vi "Test UI-Bus U32 Vars.vi"() -> ()   [LabVIEW 2021]
uses:
  Source/UI-Bus/UI-Bus.lvclass
  C:/Program Files (x86)/National Instruments/LabVIEW 2021/vi.lib/TSA/Omni-Bus/Omni-Bus/Bus Access/Bus_Access.lvclass
  <vilib>/TSA/Omni-Bus/Omni-Bus/Omni_Bus.lvclass
  <vilib>/TSA/Omni-Bus/Omni-Bus/Support/Broad Types.ctl
  <vilib>/Utility/Data Type/Type Definitions/Data Type.ctl
  <vilib>/TSA/Abstract Data Classes/Abs_Types/Type/Abs_Type.lvclass/Abs_Type.ctl
  <vilib>/TSA/Omni-Bus/Omni-Bus/Omni_Bus.lvclass/Omni_Bus.ctl
  <vilib>/TSA/Omni-Bus/Omni-Bus/Support/Read/Read Multi U32.vi
  <vilib>/TSA/Omni-Bus/Omni-Bus/Support/Write/Write U32.vi
  <vilib>/TSA/Omni-Bus/Omni-Bus/Support/Get/Get Multi U32.vi
  <vilib>/TSA/Omni-Bus/Omni-Bus/Support/FindVar.vi
  <vilib>/TSA/Omni-Bus/Omni-Bus/Support/FindMultiVar.vi
  <vilib>/Utility/error.llb/Clear Errors.vi
  <vilib>/TSA/Omni-Bus/Omni-Bus/Properties/Read Var Map.vi
  <vilib>/TSA/Abstract Data Classes/Abs_Types/Type/Properties/Read Tag.vi
  <vilib>/TSA/Abstract Data Classes/Abs_Types/U32 Integer/Abs_U32 Integer.lvclass
  C:/Program Files (x86)/National Instruments/LabVIEW 2021/vi.lib/TSA/Abstract Data Classes/Abs_Types/Type/Abs_Type.lvclass
  <vilib>/TSA/Abstract Data Classes/Abs_Types/Value/Abs_Value.lvclass
  <vilib>/TSA/Omni-Bus/Omni-Bus/Support/Check For Read Only Error.vi
  <vilib>/TSA/Omni-Bus/Omni-Bus/Support/Incorrect Tag String Error.vi
  <vilib>/TSA/Abstract Data Classes/Abs_Types/Type/Abs_Type.lvclass
  <vilib>/Utility/Data Type/NI_Data Type.lvlib
panel:
  in  "Tab Control":enum32{"Page 1", "Page 2"}(tab)
  out "Gauge":u32(knob) scale=0.0..10.0
  out "Tank":u32(slide) scale=0.0..10.0
  out "Thermometer":u32(slide) scale=0.0..100.0
  in  "Dial":u32(knob) scale=0.0..10.0
  out "Meter":u32(knob) scale=0.0..10.0
  in  "Knob":u32(knob) scale=0.0..10.0
  out "Slide 9":u32(slide) scale=0.0..100.0
  out "Slide 8":u32(slide) scale=0.0..100.0
  in  "Slide 7":u32(slide) scale=0.0..10.0
  in  "Slide 6":u32(slide) scale=0.0..10.0
  out "Slide 5":u32(slide) scale=0.0..100.0
  out "Slide 4":u32(slide) scale=0.0..100.0
  out "Slide 3":u32(slide) scale=0.0..100.0
  in  "Slide 2":u32(slide) scale=0.0..10.0
  in  "Slide":u32(slide) scale=0.0..10.0
  out "Numeric 3":u32
  in  "Numeric 2":u32
  in  "Numeric":u32
  out "U16s":u8[](array[numeric])
  in  "Tag List":string(combo)
  out "error":errorcluster
  in  "stop":bool
  out "Tags":string[](array[string])
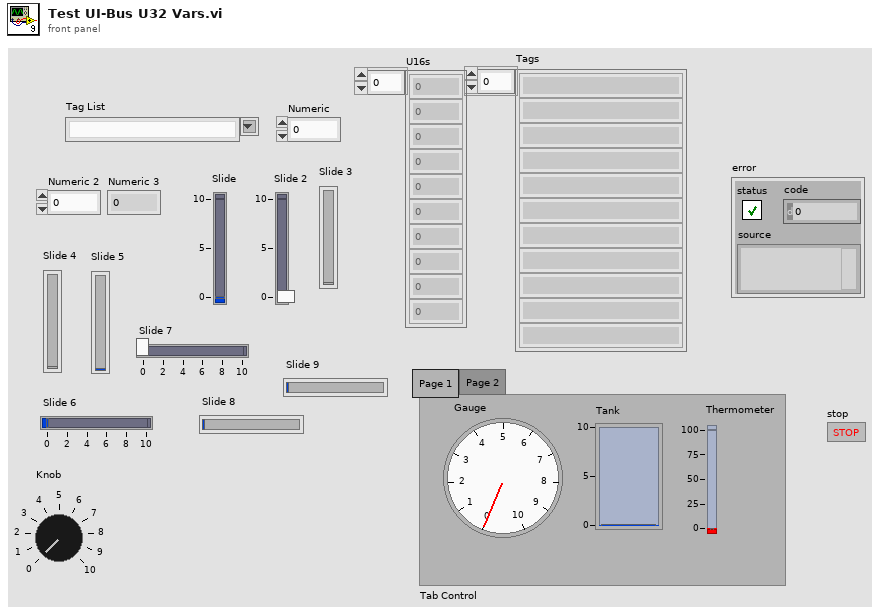
[diagram p1: front panel]
types:
  T1 = typedef "NI_Data Type.lvlib/Data Type.ctl" = enum8{"Invalid Type", "Void", "I8", "I16", "I32", "I64", "U8", "U16", "U32", "U64", "Single Float", "Double Float", "Extended Float", "Single Complex", "Double Complex", "Extended Complex", "Enum U8", "Enum U16", "Enum U32", "Enum U64", "Single Float With Unit", "Double Float With Unit", "Extended Float With Unit", "Single Complex with Unit", "Double Complex with Unit", "Extended Complex with Unit", "Boolean", "String", "Path", "Picture", "Tag", "Array", "Cluster", "Variant", "LV Variant", "Waveform", "Timestamp", "Digital Waveform", "Digital Data", "ExpressData", "Refnum", "External Data", "VI", "Poly VI", "LabVIEW Class Instance", "Fixed Point", "Set Collection", "Map Collection"}
  T2 = typedef "Omni_Bus.lvclass/Broad Types.ctl" = enum16{"All Tags", "NI Specific Type", "Boolean", "String", "Numeric", "Float", "Integer", "Collection", "All Value Types", "Non Value Types"}
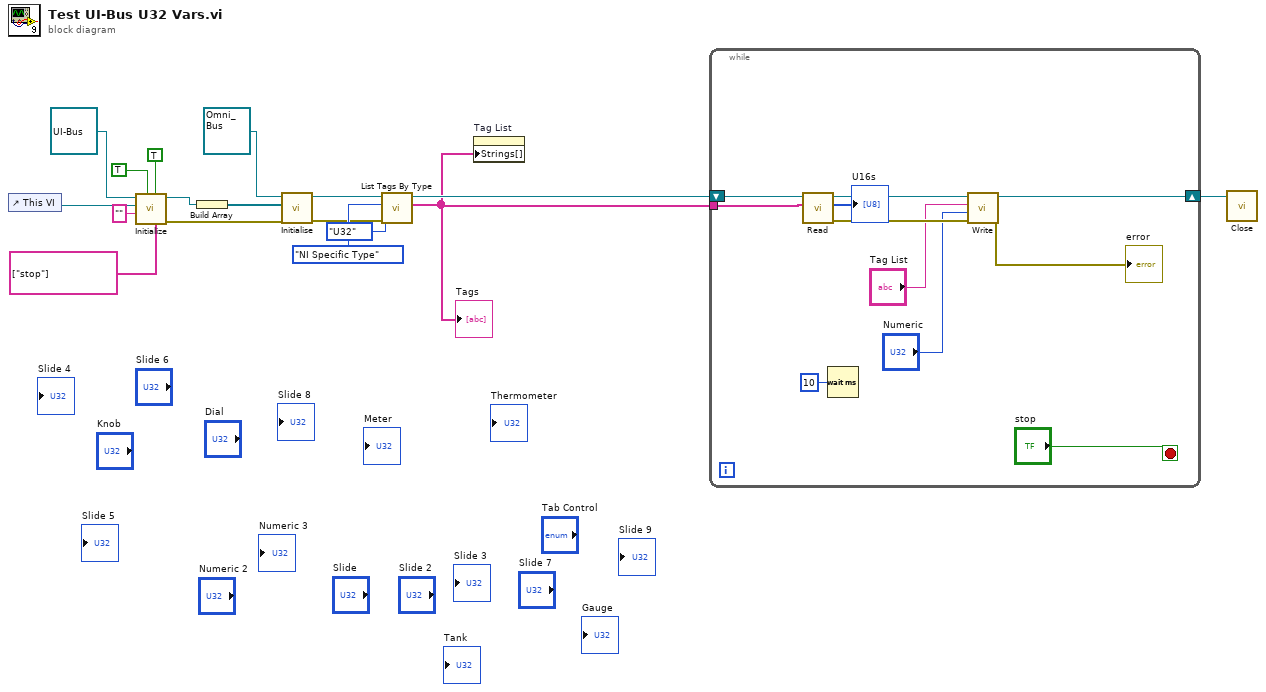
[diagram p0: block diagram]
diagram:
  n1 = control-ref of="This VI"() -> (w16:refnum<vi>)
  n2 = call "Initialize.vi"("Label Match Black List"=string[] ["stop"] ("Label Black List"), "Reset to Defaults"=TRUE, "Tab Label in Tag"=TRUE, "Tag Root"="", "VI Refnum"=w16, "UI-Bus in"=refnum<class "UI-Bus.lvclass"> refnum) -> ("error out"=w12:errorcluster, "UI-Bus out"=w14:refnum<class "UI-Bus.lvclass">)  [unwired: 4 in]
  n3 = Build Array(w14) -> (w13:refnum<class "UI-Bus.lvclass">[])
  n4 = call-dynamic "Initialise.vi"("error in (no error)"=w12, "Bus Access"=w13, "Var Bus in"=refnum<class "Omni_Bus.lvclass"> refnum) -> ("error out"=w4:errorcluster, "Var Bus out"=w5:refnum<class "Omni_Bus.lvclass">)  [unwired: 7 in]
  n5 = call <vilib>:"List Tags By Type.vi"("error in (no error)"=w4, "NI Specific Type"=Data_Type."U32", "Broad Types"=Broad_Types."NI Specific Type", "Var Bus in"=w5) -> ("Tags"=w3:string[], "Var Bus out"=w10:refnum<class "Omni_Bus.lvclass">)  [unwired: 4 in, 2 out]
  "Tags" <- w3
  n6 = property on="Tag List" class="CmbBox"("Strings[]"=w3) -> ()  [unwired: 2 in, 2 out]
  n7 = while {
    tunnel: w3 -> [w28]
    shift-right: [w22] -> w9
    shift-left: w10 -> [w27]
    stop <- "stop" stop-if-true
    n8 = call-poly <vilib>:"Read.vi"("Tag"=w28, "Var Bus in"=w27) -> ("error out"=w23:errorcluster, "U32's"=→"U16s":u32[], "Var Bus out"=w24:refnum<class "Omni_Bus.lvclass">)  [unwired: 7 in]
    n9 = Wait (ms)(milliseconds to wait=u32 10) -> ()  [unwired: 1 out]
    n10 = call-poly <vilib>:"Write.vi"("error in (no error)"=w23, "Numeric"="Numeric", "Tag"="Tag List", "Omni_Bus in"=w24) -> ("error out"=→"error":errorcluster, "Omni_Bus out"=w22:refnum<class "Omni_Bus.lvclass">)  [unwired: 6 in]
  }
  n11 = call-dynamic "Close.vi"("Data in"=w9) -> ()  [unwired: 9 in, 2 out]
